vi "InitDrive.vi"   [LabVIEW 2019]
uses:
  <vilib>/Rock Robotics/WPI/ThirdParty/REV Robotics/SPARK MAX/Typedef/Spark MAX Idle Mode.ctl
  refnums.vi
  <vilib>/Rock Robotics/WPI/MotorControl/WPI_MotorControlOpen SPARK_MAX.vi
  <vilib>/Rock Robotics/SystemInterfaces/DIO/FPGA_DIOPWMChannel.ctl
types:
  T1 = typedef "Spark MAX Idle Mode.ctl" = enum16{"Coast", "Brake"}
  T2 = typedef "FPGA_DIOPWMChannel.ctl" = enum8{"PWM 0", "PWM 1", "PWM 2", "PWM 3", "PWM 4", "PWM 5", "PWM 6", "PWM 7", "PWM 8", "PWM 9", "PWM MXP 0", "PWM MXP 1", "PWM MXP 2", "PWM MXP 3", "PWM MXP 4", "PWM MXP 5", "PWM MXP 6", "PWM MXP 7", "PWM MXP 8", "PWM MXP 9", "Invalid"}
  T3 = typedef "WPI_MotorControlDeviceRef.ctl" = cluster{"DeviceStatus":errorcluster, "Type":T4, "PWM":cluster{"PWM Channel":T2, "DeadBand":T5}, "CAN":cluster{"Device Number":u8, "SetOutput VI Ref":variant, "GetOutput VI Ref":variant, "Enable VI Ref":variant, "Disable VI Ref":variant, "Data":variant}, "Invert":bool, "DIO PWM":cluster{"PWM \"Enable\" Channel":T2, "DIOChannel":T6, "PWM Rate":dbl}}
  T4 = typedef "WPI_MotorControlType.ctl" = enum16{"PWM", "CAN", "DIO PWM"}
  T5 = typedef "WPI_PWMDeadband.ctl" = cluster{"Name":string, "maxPositivePwm":i32, "minPositivePwm":i32, "centerPwm":i32, "maxNegativePwm":i32, "minNegativePwm":i32, "angularRange":u16}
  T6 = typedef "FPGA_DIOChannel.ctl" = enum8{"DIO 0", "DIO 1", "DIO 2", "DIO 3", "DIO 4", "DIO 5", "DIO 6", "DIO 7", "DIO 8", "DIO 9", "DIO MXP 0", "DIO MXP 1", "DIO MXP 2", "DIO MXP 3", "DIO MXP 4", "DIO MXP 5", "DIO MXP 6", "DIO MXP 7", "DIO MXP 8", "DIO MXP 9", "DIO MXP 10", "DIO MXP 11", "DIO MXP 12", "DIO MXP 13", "DIO MXP 14", "DIO MXP 15", "SPI Port CS1", "SPI Port CS2", "SPI Port CS3", "SPI Port MISO", "SPI Port MOSI", "Invalid"}
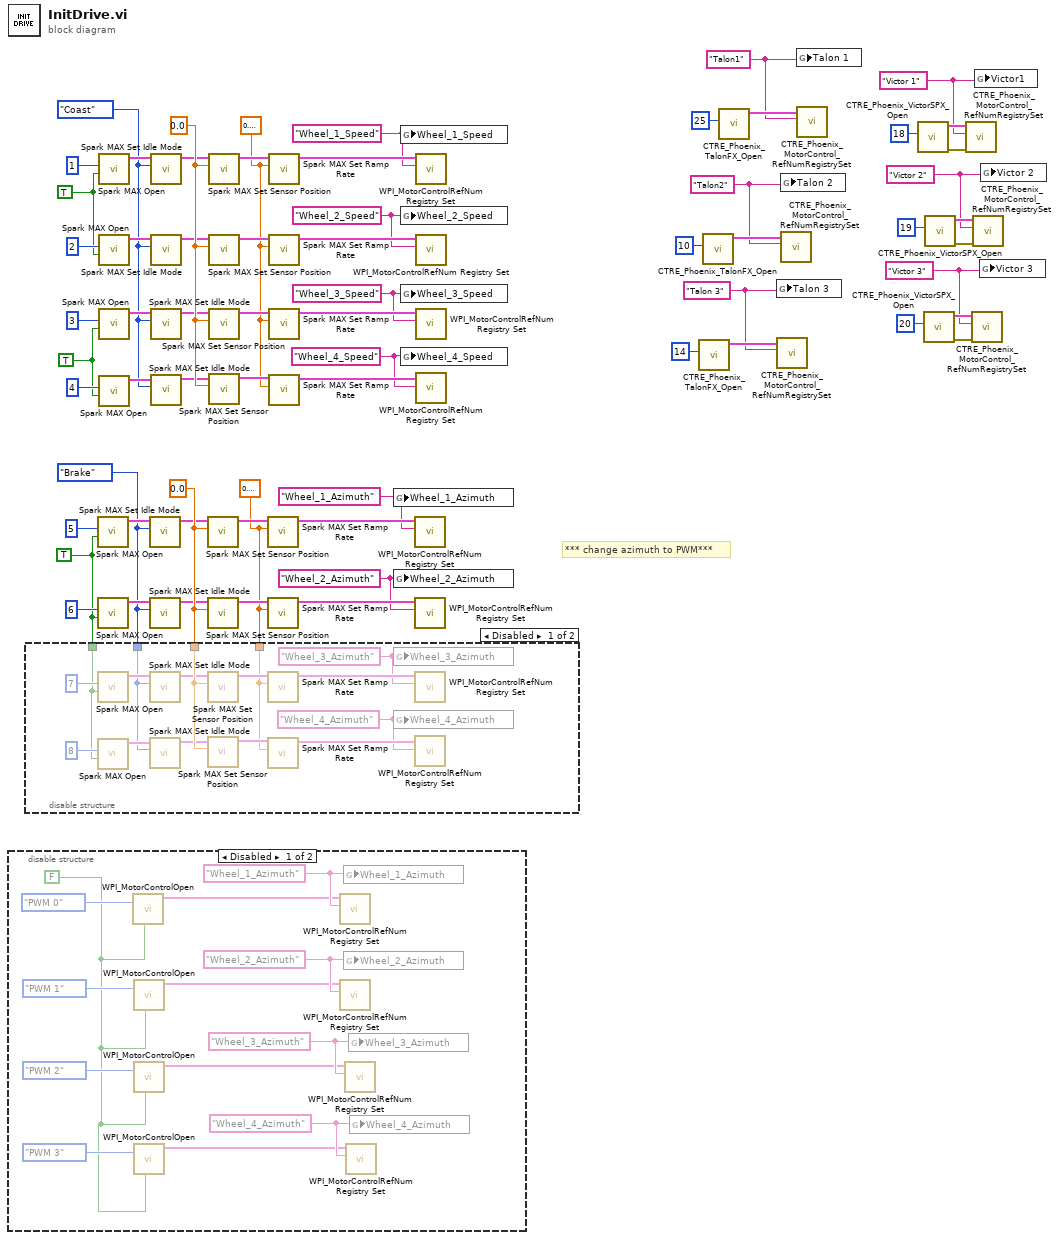
[diagram p0: block diagram]
diagram:
  w4 = "Victor 3" ("refnum name")
  w7 = "Victor 2" ("refnum name")
  w10 = "Victor 1" ("refnum name")
  w13 = "Talon 3" ("refnum name")
  w16 = "Talon2" ("refnum name")
  w19 = "Talon1" ("refnum name")
  w22 = TRUE
  w38 = 0.0
  w24 = TRUE
  w25 = "Wheel_2_Azimuth" ("refnum name")
  w23 = Spark_MAX_Idle_Mode."Brake" ("Idle Mode")
  w26 = "Wheel_1_Azimuth" ("refnum name")
  w27 = sgl 0.1 ("Seconds from neutral to full (0)")
  w66 = 0.0
  w40 = TRUE
  w42 = "Wheel_3_Speed" ("refnum name")
  w41 = "Wheel_4_Speed" ("refnum name")
  w43 = "Wheel_2_Speed" ("refnum name")
  w39 = Spark_MAX_Idle_Mode."Coast" ("Idle Mode")
  w44 = "Wheel_1_Speed" ("refnum name")
  w45 = sgl 0.2 ("Seconds from neutral to full (0)")
  # "*** change azimuth to PWM***"
  n1 = disable-structure shown="Disabled" {
    frame Disabled {
      w68 = "Wheel_4_Azimuth" ("refnum name")
      w70 = "Wheel_3_Azimuth" ("refnum name")
      w72 = "Wheel_2_Azimuth" ("refnum name")
      w74 = "Wheel_1_Azimuth" ("refnum name")
      w75 = FALSE ("Invert")
      n2 = call-poly <vilib>:"WPI_MotorControlOpen.vi"("Invert"=w75, "PWM Channel"=FPGA_DIOPWMChannel."PWM 0") -> ("MotorControlDeviceRef"=w73:T3)  [unwired: 8 in, 1 out]
      n3 = call-poly <vilib>:"WPI_MotorControlOpen.vi"("Invert"=w75, "PWM Channel"=FPGA_DIOPWMChannel."PWM 1") -> ("MotorControlDeviceRef"=w71:T3)  [unwired: 8 in, 1 out]
      n4 = call-poly <vilib>:"WPI_MotorControlOpen.vi"("Invert"=w75, "PWM Channel"=FPGA_DIOPWMChannel."PWM 2") -> ("MotorControlDeviceRef"=w69:T3)  [unwired: 8 in, 1 out]
      n5 = call-poly <vilib>:"WPI_MotorControlOpen.vi"("Invert"=w75, "PWM Channel"=FPGA_DIOPWMChannel."PWM 3") -> ("MotorControlDeviceRef"=w67:T3)  [unwired: 8 in, 1 out]
      n6 = call <vilib>:"WPI_MotorControlRefNum Registry Set.vi"("refnum name"=w74, "MotorControlDevRef"=w73) -> ()  [unwired: 8 in, 2 out]
      n7 = call <vilib>:"WPI_MotorControlRefNum Registry Set.vi"("refnum name"=w72, "MotorControlDevRef"=w71) -> ()  [unwired: 8 in, 2 out]
      n8 = global write "refnums.vi" "Wheel_1_Azimuth"(w74) -> ()
      n9 = global write "refnums.vi" "Wheel_2_Azimuth"(w72) -> ()
      n10 = call <vilib>:"WPI_MotorControlRefNum Registry Set.vi"("refnum name"=w70, "MotorControlDevRef"=w69) -> ()  [unwired: 8 in, 2 out]
      n11 = call <vilib>:"WPI_MotorControlRefNum Registry Set.vi"("refnum name"=w68, "MotorControlDevRef"=w67) -> ()  [unwired: 8 in, 2 out]
      n12 = global write "refnums.vi" "Wheel_3_Azimuth"(w70) -> ()
      n13 = global write "refnums.vi" "Wheel_4_Azimuth"(w68) -> ()
    }
    frame Enabled {
    }
  }
  n14 = disable-structure shown="Disabled" {
    disable-tunnel: w38 -> [w95 _]
    disable-tunnel: w27 -> [w84 _]
    disable-tunnel: w24 -> [w81 _]
    disable-tunnel: w23 -> [w80 _]
    frame Disabled {
      w83 = "Wheel_3_Azimuth" ("refnum name")
      w82 = "Wheel_4_Azimuth" ("refnum name")
      n15 = call <vilib>:"Spark MAX Open.vi"("Invert"=w81, "Device Number"=u8 7 ("Drive  3R")) -> ("MotorControlDeviceRef"=w88:T3)  [unwired: 8 in, 1 out]
      n16 = call <vilib>:"Spark MAX Open.vi"("Invert"=w81, "Device Number"=u8 8 ("Drive 4L")) -> ("MotorControlDeviceRef"=w85:T3)  [unwired: 8 in, 1 out]
      n17 = call <vilib>:"Spark MAX Set Idle Mode.vi"("Idle Mode"=w80, "MotorControlDeviceRef in"=w88) -> ("MotorControlDeviceRef out"=w91:T3)  [unwired: 8 in, 1 out]
      n18 = call <vilib>:"Spark MAX Set Idle Mode.vi"("Idle Mode"=w80, "MotorControlDeviceRef in"=w85) -> ("MotorControlDeviceRef out"=w93:T3)  [unwired: 8 in, 1 out]
      n19 = call <vilib>:"Spark MAX Set Sensor Position.vi"("Position"=w95, "MotorControlDeviceRef"=w91) -> ("MotorControlDeviceRef"=w92:T3)  [unwired: 8 in, 1 out]
      n20 = call <vilib>:"Spark MAX Set Sensor Position.vi"("Position"=w95, "MotorControlDeviceRef"=w93) -> ("MotorControlDeviceRef"=w94:T3)  [unwired: 8 in, 1 out]
      n21 = call <vilib>:"Spark MAX Set Ramp Rate.vi"("Seconds from neutral to full (0)"=w84, "MotorControlDeviceRef in"=w92) -> ("MotorControlDeviceRef"=w90:T3)  [unwired: 8 in, 1 out]
      n22 = call <vilib>:"Spark MAX Set Ramp Rate.vi"("Seconds from neutral to full (0)"=w84, "MotorControlDeviceRef in"=w94) -> ("MotorControlDeviceRef"=w87:T3)  [unwired: 8 in, 1 out]
      n23 = global write "refnums.vi" "Wheel_3_Azimuth"(w83) -> ()
      n24 = global write "refnums.vi" "Wheel_4_Azimuth"(w82) -> ()
      n25 = call <vilib>:"WPI_MotorControlRefNum Registry Set.vi"("refnum name"=w83, "MotorControlDevRef"=w90) -> ()  [unwired: 8 in, 2 out]
      n26 = call <vilib>:"WPI_MotorControlRefNum Registry Set.vi"("refnum name"=w82, "MotorControlDevRef"=w87) -> ()  [unwired: 8 in, 2 out]
    }
    frame Enabled {
    }
  }
  n27 = call <vilib>:"Spark MAX Open.vi"("Invert"=w24, "Device Number"=u8 5 ("Drive 1R")) -> ("MotorControlDeviceRef"=w28:T3)  [unwired: 8 in, 1 out]
  n28 = call <vilib>:"Spark MAX Open.vi"("Invert"=w24, "Device Number"=u8 6 ("Drive 2R")) -> ("MotorControlDeviceRef"=w31:T3)  [unwired: 8 in, 1 out]
  n29 = call <vilib>:"Spark MAX Open.vi"("Invert"=w40, "Device Number"=u8 1 ("Drive 1R")) -> ("MotorControlDeviceRef"=w46:T3)  [unwired: 8 in, 1 out]
  n30 = call <vilib>:"Spark MAX Open.vi"("Invert"=w40, "Device Number"=u8 2 ("Drive 2R")) -> ("MotorControlDeviceRef"=w49:T3)  [unwired: 8 in, 1 out]
  n31 = call <vilib>:"Spark MAX Open.vi"("Invert"=w22, "Device Number"=u8 3 ("Drive  3R")) -> ("MotorControlDeviceRef"=w55:T3)  [unwired: 8 in, 1 out]
  n32 = call <vilib>:"Spark MAX Open.vi"("Invert"=w22, "Device Number"=u8 4 ("Drive 4L")) -> ("MotorControlDeviceRef"=w52:T3)  [unwired: 8 in, 1 out]
  n33 = call <vilib>:"Spark MAX Set Idle Mode.vi"("Idle Mode"=w23, "MotorControlDeviceRef in"=w28) -> ("MotorControlDeviceRef out"=w34:T3)  [unwired: 8 in, 1 out]
  n34 = call <vilib>:"Spark MAX Set Idle Mode.vi"("Idle Mode"=w23, "MotorControlDeviceRef in"=w31) -> ("MotorControlDeviceRef out"=w36:T3)  [unwired: 8 in, 1 out]
  n35 = call <vilib>:"Spark MAX Set Idle Mode.vi"("Idle Mode"=w39, "MotorControlDeviceRef in"=w46) -> ("MotorControlDeviceRef out"=w58:T3)  [unwired: 8 in, 1 out]
  n36 = call <vilib>:"Spark MAX Set Idle Mode.vi"("Idle Mode"=w39, "MotorControlDeviceRef in"=w49) -> ("MotorControlDeviceRef out"=w60:T3)  [unwired: 8 in, 1 out]
  n37 = call <vilib>:"Spark MAX Set Idle Mode.vi"("Idle Mode"=w39, "MotorControlDeviceRef in"=w55) -> ("MotorControlDeviceRef out"=w62:T3)  [unwired: 8 in, 1 out]
  n38 = call <vilib>:"Spark MAX Set Idle Mode.vi"("Idle Mode"=w39, "MotorControlDeviceRef in"=w52) -> ("MotorControlDeviceRef out"=w64:T3)  [unwired: 8 in, 1 out]
  n39 = call <vilib>:"Spark MAX Set Sensor Position.vi"("Position"=w38, "MotorControlDeviceRef"=w34) -> ("MotorControlDeviceRef"=w35:T3)  [unwired: 8 in, 1 out]
  n40 = call <vilib>:"Spark MAX Set Sensor Position.vi"("Position"=w38, "MotorControlDeviceRef"=w36) -> ("MotorControlDeviceRef"=w37:T3)  [unwired: 8 in, 1 out]
  n41 = call <vilib>:"Spark MAX Set Sensor Position.vi"("Position"=w66, "MotorControlDeviceRef"=w58) -> ("MotorControlDeviceRef"=w59:T3)  [unwired: 8 in, 1 out]
  n42 = call <vilib>:"Spark MAX Set Sensor Position.vi"("Position"=w66, "MotorControlDeviceRef"=w60) -> ("MotorControlDeviceRef"=w61:T3)  [unwired: 8 in, 1 out]
  n43 = call <vilib>:"Spark MAX Set Sensor Position.vi"("Position"=w66, "MotorControlDeviceRef"=w62) -> ("MotorControlDeviceRef"=w63:T3)  [unwired: 8 in, 1 out]
  n44 = call <vilib>:"Spark MAX Set Sensor Position.vi"("Position"=w66, "MotorControlDeviceRef"=w64) -> ("MotorControlDeviceRef"=w65:T3)  [unwired: 8 in, 1 out]
  n45 = call <vilib>:"Spark MAX Set Ramp Rate.vi"("Seconds from neutral to full (0)"=w27, "MotorControlDeviceRef in"=w35) -> ("MotorControlDeviceRef"=w29:T3)  [unwired: 8 in, 1 out]
  n46 = call <vilib>:"Spark MAX Set Ramp Rate.vi"("Seconds from neutral to full (0)"=w27, "MotorControlDeviceRef in"=w37) -> ("MotorControlDeviceRef"=w33:T3)  [unwired: 8 in, 1 out]
  n47 = call <vilib>:"Spark MAX Set Ramp Rate.vi"("Seconds from neutral to full (0)"=w45, "MotorControlDeviceRef in"=w59) -> ("MotorControlDeviceRef"=w47:T3)  [unwired: 8 in, 1 out]
  n48 = call <vilib>:"Spark MAX Set Ramp Rate.vi"("Seconds from neutral to full (0)"=w45, "MotorControlDeviceRef in"=w61) -> ("MotorControlDeviceRef"=w51:T3)  [unwired: 8 in, 1 out]
  n49 = call <vilib>:"Spark MAX Set Ramp Rate.vi"("Seconds from neutral to full (0)"=w45, "MotorControlDeviceRef in"=w63) -> ("MotorControlDeviceRef"=w57:T3)  [unwired: 8 in, 1 out]
  n50 = call <vilib>:"Spark MAX Set Ramp Rate.vi"("Seconds from neutral to full (0)"=w45, "MotorControlDeviceRef in"=w65) -> ("MotorControlDeviceRef"=w54:T3)  [unwired: 8 in, 1 out]
  n51 = global write "refnums.vi" "Wheel_1_Azimuth"(w26) -> ()
  n52 = global write "refnums.vi" "Wheel_2_Azimuth"(w25) -> ()
  n53 = global write "refnums.vi" "Wheel_1_Speed"(w44) -> ()
  n54 = global write "refnums.vi" "Wheel_2_Speed"(w43) -> ()
  n55 = global write "refnums.vi" "Wheel_3_Speed"(w42) -> ()
  n56 = global write "refnums.vi" "Wheel_4_Speed"(w41) -> ()
  n57 = call <vilib>:"WPI_MotorControlRefNum Registry Set.vi"("refnum name"=w26, "MotorControlDevRef"=w29) -> ()  [unwired: 8 in, 2 out]
  n58 = call <vilib>:"WPI_MotorControlRefNum Registry Set.vi"("refnum name"=w25, "MotorControlDevRef"=w33) -> ()  [unwired: 8 in, 2 out]
  n59 = call <vilib>:"WPI_MotorControlRefNum Registry Set.vi"("refnum name"=w44, "MotorControlDevRef"=w47) -> ()  [unwired: 8 in, 2 out]
  n60 = call <vilib>:"WPI_MotorControlRefNum Registry Set.vi"("refnum name"=w43, "MotorControlDevRef"=w51) -> ()  [unwired: 8 in, 2 out]
  n61 = call <vilib>:"WPI_MotorControlRefNum Registry Set.vi"("refnum name"=w42, "MotorControlDevRef"=w57) -> ()  [unwired: 8 in, 2 out]
  n62 = call <vilib>:"WPI_MotorControlRefNum Registry Set.vi"("refnum name"=w41, "MotorControlDevRef"=w54) -> ()  [unwired: 8 in, 2 out]
  n63 = call <vilib>:"CTRE_Phoenix_TalonFX_Open.vi"("Device Number"=u8 14) -> ("CAN Talon SRX Ref"=w14:T3)  [unwired: 9 in, 1 out]
  n64 = call <vilib>:"CTRE_Phoenix_TalonFX_Open.vi"("Device Number"=u8 10) -> ("CAN Talon SRX Ref"=w17:T3)  [unwired: 9 in, 1 out]
  n65 = call <vilib>:"CTRE_Phoenix_TalonFX_Open.vi"("Device Number"=u8 25) -> ("CAN Talon SRX Ref"=w20:T3)  [unwired: 9 in, 1 out]
  n66 = global write "refnums.vi" "Talon 3"(w13) -> ()
  n67 = call <vilib>:"CTRE_Phoenix_MotorControl_RefNumRegistrySet.vi"("refnum name"=w13, "PhoenixMotorControlDevRef"=w14) -> ()  [unwired: 8 in, 2 out]
  n68 = global write "refnums.vi" "Talon 2"(w16) -> ()
  n69 = call <vilib>:"CTRE_Phoenix_MotorControl_RefNumRegistrySet.vi"("refnum name"=w16, "PhoenixMotorControlDevRef"=w17) -> ()  [unwired: 8 in, 2 out]
  n70 = global write "refnums.vi" "Talon 1"(w19) -> ()
  n71 = call <vilib>:"CTRE_Phoenix_MotorControl_RefNumRegistrySet.vi"("refnum name"=w19, "PhoenixMotorControlDevRef"=w20) -> ()  [unwired: 8 in, 2 out]
  n72 = call <vilib>:"CTRE_Phoenix_VictorSPX_Open.vi"("Device Number"=u8 18) -> ("error out"=w12:errorcluster, "CAN Talon SRX Ref"=w11:T3)  [unwired: 9 in]
  n73 = call <vilib>:"CTRE_Phoenix_VictorSPX_Open.vi"("Device Number"=u8 20) -> ("error out"=w6:errorcluster, "CAN Talon SRX Ref"=w5:T3)  [unwired: 9 in]
  n74 = call <vilib>:"CTRE_Phoenix_VictorSPX_Open.vi"("Device Number"=u8 19) -> ("error out"=w9:errorcluster, "CAN Talon SRX Ref"=w8:T3)  [unwired: 9 in]
  n75 = call <vilib>:"CTRE_Phoenix_MotorControl_RefNumRegistrySet.vi"("error in (no error)"=w12, "refnum name"=w10, "PhoenixMotorControlDevRef"=w11) -> ()  [unwired: 7 in, 2 out]
  n76 = call <vilib>:"CTRE_Phoenix_MotorControl_RefNumRegistrySet.vi"("error in (no error)"=w6, "refnum name"=w4, "PhoenixMotorControlDevRef"=w5) -> ()  [unwired: 7 in, 2 out]
  n77 = call <vilib>:"CTRE_Phoenix_MotorControl_RefNumRegistrySet.vi"("error in (no error)"=w9, "refnum name"=w7, "PhoenixMotorControlDevRef"=w8) -> ()  [unwired: 7 in, 2 out]
  n78 = global write "refnums.vi" "Victor1"(w10) -> ()
  n79 = global write "refnums.vi" "Victor 3"(w4) -> ()
  n80 = global write "refnums.vi" "Victor 2"(w7) -> ()
